vi "Method.vi"(8 "error in (no error)":errorcluster, 11 "Driver Project in":refnum<class "Driver Project.lvclass">) -> (0 "error out":errorcluster, 3 "Driver Project out":refnum<class "Driver Project.lvclass">)   [LabVIEW 2020, in "Driver Project.lvlib" / "Driver Project.lvclass"]
doc: "Driver template method for dynamic dispatch."
uses:
  Driver Project.lvclass
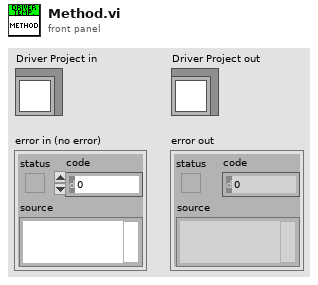
[diagram p1: front panel]
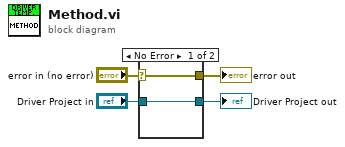
[diagram p0: block diagram]
diagram:
  n1 = case shown="No Error" "error in (no error)" {
    selector: "error in (no error)" -> [w5 w8]
    tunnel: [w5 w8] -> w3
    tunnel: [w6 w7] -> w1
    tunnel: "Driver Project in" -> [w6 w7]
    frame No Error {
    }
    frame Error {
    }
  }
  "error out" <- w3
  "Driver Project out" <- w1
